vi "20220105_ArbitraryWaveGenDAQ.vi"() -> ()   [LabVIEW 2021]
uses:
  <vilib>/DAQmx/write.llb/DAQmx Write (Analog Wfm 1Chan NSamp).vi
  <vilib>/DAQmx/create/channels.llb/DAQmx Create Channel (AO-Voltage-Basic).vi
  <vilib>/DAQmx/configure/timing.llb/DAQmx Timing (Sample Clock).vi
  <vilib>/Utility/file.llb/Read Delimited Spreadsheet (DBL).vi
  <vilib>/DAQmx/miscellaneous.llb/DAQmx Fill In Error Info.vi
  <vilib>/Analysis/NI_AALBase.lvlib
panel:
  in  "DataColumn":i32
  in  "Frequency Unit":u16(ring) items=["Hz", "cycles"]
  in  "Stop":bool
  in  "Reset phase":bool
  in  "Sampling rate (Hz)":dbl=100.0 step=1.0 format="%#.3g"
  in  "Frequency":dbl=2.01 step=1.0 format="%0.2f"
  out "Waveform Pattern":dbl[](graph)
  out "Signal Generated":T1(graph)={0.0, 0.01, "arbitrary wave"=[]}
  in  "interpolation":i32(ring)=1 items=["none", "linear"]
  in  "Amplitude":dbl(slide)=3.7755102040816326 scale=0.0..5.0
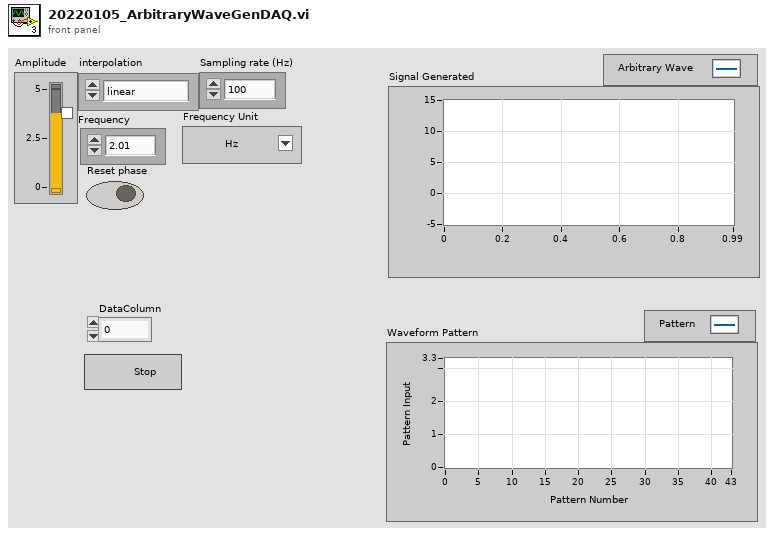
[diagram p1: front panel]
types:
  T1 = cluster{dbl[unit], dbl[unit], "arbitrary wave":dbl[]}
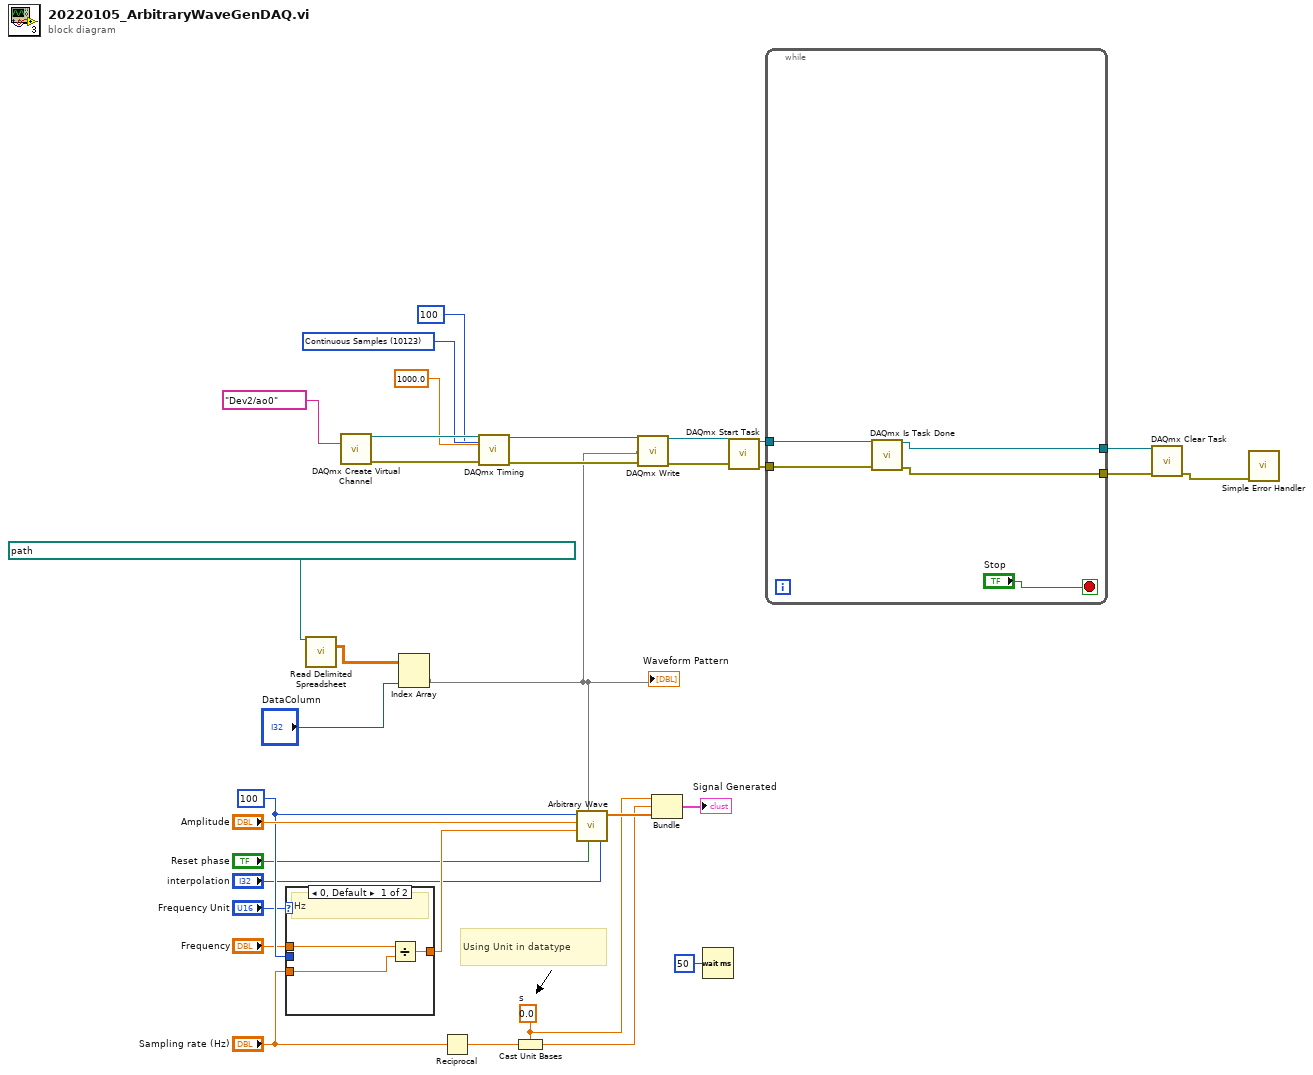
[diagram p0: block diagram]
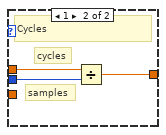
[diagram p2: hidden frame]
diagram:
  w13 = dbl[unit] 0.0  # s
  w23 = 100 ("samples")
  w29 = 10123 items=["Finite Samples"=10178, "Continuous Samples"=10123, "Hardware Timed Single Point"=12522] ("sample mode")
  # "Using Unit in datatype"
  n1 = case shown="0, Default" "Frequency Unit" {
    tunnel: [w36 w38] -> w24
    tunnel: w23 -> [_ w39]
    tunnel: "Frequency" -> [w35 w37]
    tunnel: "Sampling rate (Hz)" -> [w34 _]
    frame 0, Default {
      # "Hz"
      n2 = Divide(x=w35, y=w34) -> (x/y=w36:dbl)
    }
    frame 1 {
      # "samples"
      # "cycles"
      # "Cycles"
      n3 = Divide(x=w37, y=w39) -> (x/y=w38:dbl)
    }
  }
  n4 = call-poly <vilib>:"Read Delimited Spreadsheet.vi"("file path (dialog if empty)"=path "C:/Users/joe.kao/OneDrive - eCloudvalley Digital Technology/桌面/nPM1100_Muon_Waveform.txt") -> ("all rows"=w10:dbl[][])  [unwired: 9 in, 5 out]
  n5 = call-poly <vilib>:"DAQmx Create Virtual Channel.vi"("physical channels"=tag "Dev2/ao0") -> ("task out"=w32:refnum<k21>, "error out"=w31:errorcluster)  [unwired: 13 in]
  n6 = Index Array(array=w10, index (col)="DataColumn") -> (element=w9:dbl[])  [unwired: 1 in]
  "Waveform Pattern" <- w9
  n7 = Reciprocal(x="Sampling rate (Hz)") -> (1/x=w17:dbl)
  n8 = call-poly <vilib>:"DAQmx Timing.vi"("task/channels in"=w32, "sample mode"=w29, "samples per channel"=100, "rate"=1000.0, "error in"=w31) -> ("task out"=w27:refnum<k21>, "error out"=w26:errorcluster)  [unwired: 9 in]
  n9 = Cast Unit Bases(0:w17, 1:w13) -> (2:w16:dbl[unit])
  n10 = call <vilib>:"Arbitrary Wave.vi"("interpolation"="interpolation", "reset phase"="Reset phase", "Wave Table"=w9, "frequency"=w24, "amplitude"="Amplitude", "samples"=w23) -> ("arbitrary wave"=w19:dbl[])  [unwired: 1 in, 2 out]
  n11 = call-poly <vilib>:"DAQmx Write.vi"("task/channels in"=w27, "data"=w9, "error in"=w26) -> ("task out"=w8:refnum<k21>, "error out"=w7:errorcluster)  [unwired: 10 in, 1 out]
  n12 = Bundle(w13, w16, "arbitrary wave"=w19) -> (→"Signal Generated":T1)  [unwired: 1 in]
  n13 = Wait (ms)(milliseconds to wait=u32 50) -> ()  [unwired: 1 out]
  n14 = call <vilib>:"DAQmx Start Task.vi"("task/channels in"=w8, "error in"=w7) -> ("task out"=w6:refnum<k21>, "error out"=w5:errorcluster)  [unwired: 12 in]
  n15 = while {
    tunnel: w6 -> [w43]
    tunnel: w5 -> [w42]
    tunnel: [w41] -> w4
    tunnel: [w40] -> w3
    stop <- "Stop" stop-if-true
    n16 = call <vilib>:"DAQmx Is Task Done.vi"("task/channels in"=w43, "error in"=w42) -> ("task out"=w41:refnum<k21>, "error out"=w40:errorcluster)  [unwired: 11 in, 1 out]
  }
  n17 = call <vilib>:"DAQmx Clear Task.vi"("task in"=w4, "error in"=w3) -> ("error out"=w2:errorcluster)  [unwired: 13 in]
  n18 = call <vilib>:"Simple Error Handler.vi"("error in (no error)"=w2) -> ()  [unwired: 4 in, 5 out]
